vi "ProgressControl.vi"(0 "Elapsed time IN":dbl, 1 "SP IN":dbl, 2 "Array IN":dbl[](array[numeric]), 3 "Current SP IN":dbl, 4 "Stable":bool, 5 "Initial ramp IN":bool, 6 "SP reached IN":bool, 7 "Oven Watlows":refnum<visa-resource-name>="COM4", 8 "Progress":string, 9 "Sample":dbl) -> (12 "Array":dbl[](array[numeric]), 14 "Progress":string, 15 "Current SP":dbl, 16 "Stable":bool, 17 "Initial ramp":bool, 18 "SP reached":bool)   [LabVIEW 2009]
panel:
  # "INPUT"
  # "OUTPUT"
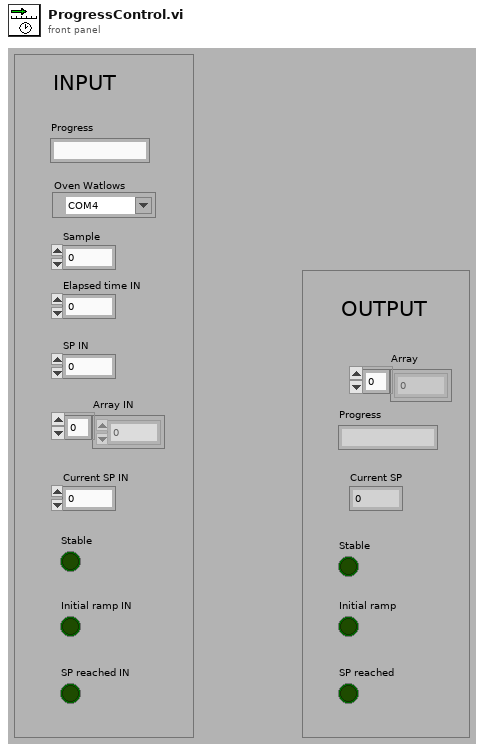
[diagram p1: front panel]
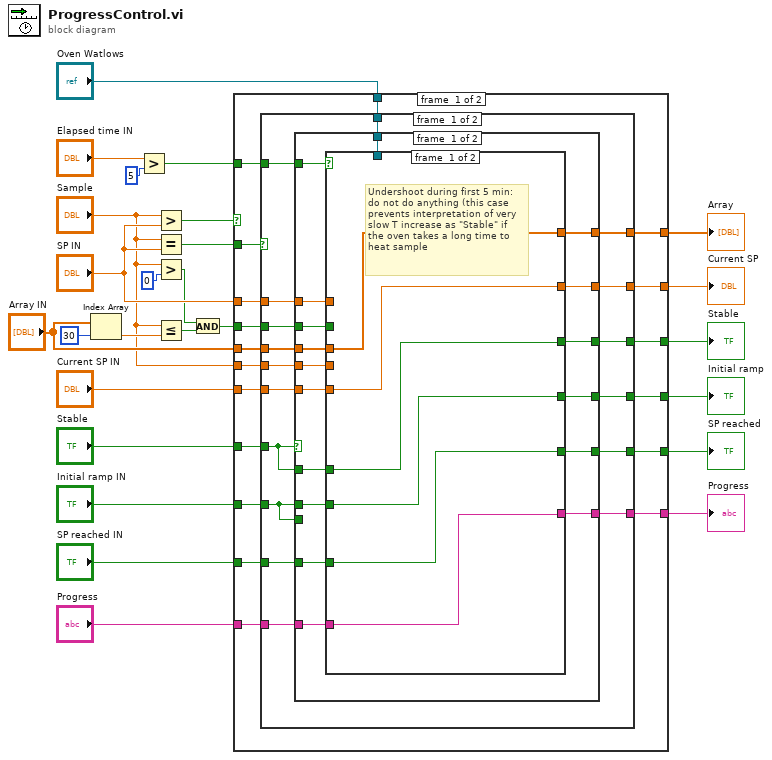
[diagram p0: block diagram]
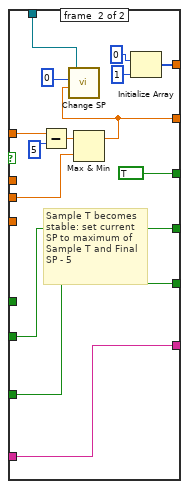
[diagram p3: hidden frame]
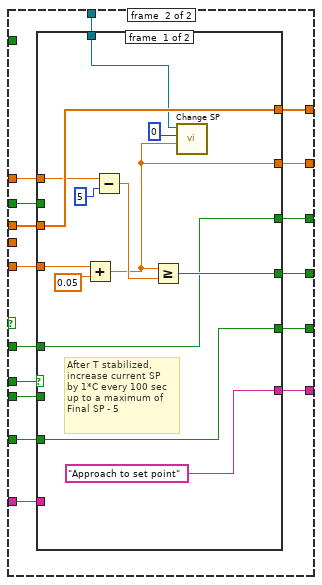
[diagram p4: hidden frame]
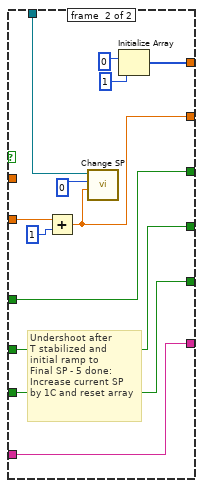
[diagram p6: hidden frame]
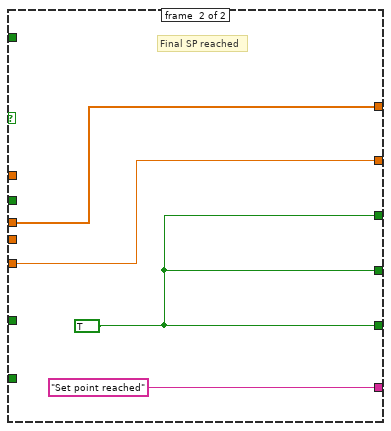
[diagram p7: hidden frame]
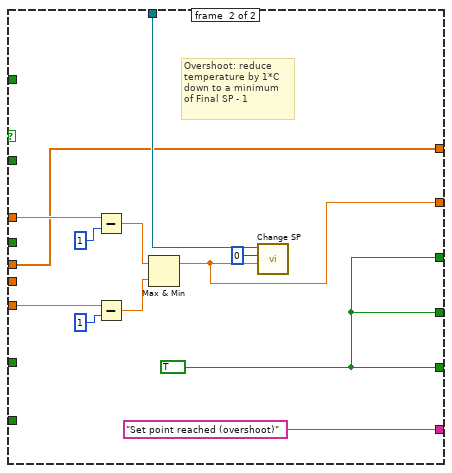
[diagram p8: hidden frame]
diagram:
  n1 = Index Array(array="Array IN", index=30) -> (element=w19:dbl)
  n2 = Greater?(x="Elapsed time IN", y=5) -> (0:w23:bool)
  n3 = Greater?(x="Sample", y="SP IN") -> (0:w6:bool)
  n4 = Equal?(x="Sample", y="SP IN") -> (x = y?=w7:bool)
  n5 = Greater?(x="Sample", y=0) -> (0:w1:bool)
  n6 = Less Or Equal?(x="Sample", y=w19) -> (x <= y?=w2:bool)
  n7 = And(x=w1, y=w2) -> (x .and. y?=w3:bool)
  n8 = case shown="False" w6 {
    tunnel: "SP reached IN" -> [w44 _]
    tunnel: w23 -> [w43 _]
    tunnel: w3 -> [w42 _]
    tunnel: "Oven Watlows" -> [w41 w188]
    tunnel: [w40 w187] -> w21
    tunnel: [w39 w186] -> w18
    tunnel: [w38 w197] -> w17
    tunnel: [w37 w197] -> w16
    tunnel: [w36 w197] -> w15
    tunnel: "Current SP IN" -> [w35 w194]
    tunnel: [w34 "Set point reached (overshoot)"] -> w13
    tunnel: "Stable" -> [w33 _]
    tunnel: "Initial ramp IN" -> [w32 _]
    tunnel: "Progress" -> [w31 _]
    tunnel: "Array IN" -> [w30 w186]
    tunnel: "Sample" -> [w29 _]
    tunnel: "SP IN" -> [w28 w191]
    tunnel: w7 -> [w27 _]
    frame #0 {
      n9 = case shown="False" w27 {
        tunnel: w44 -> [w61 _]
        tunnel: w43 -> [w60 _]
        tunnel: w42 -> [w59 _]
        tunnel: w41 -> [w58 _]
        tunnel: [w57 w183] -> w40
        tunnel: [w56 w184] -> w39
        tunnel: [w55 w182] -> w38
        tunnel: [w54 w182] -> w37
        tunnel: [w53 w182] -> w36
        tunnel: w35 -> [w52 w183]
        tunnel: [w51 "Set point reached"] -> w34
        tunnel: w33 -> [w50 _]
        tunnel: w32 -> [w49 _]
        tunnel: w31 -> [w48 _]
        tunnel: w30 -> [w47 w184]
        tunnel: w29 -> [w46 _]
        tunnel: w28 -> [w45 _]
        frame #0 {
          n10 = case shown="True" w50 {
            tunnel: w49 -> [w70 w136]
            tunnel: w61 -> [w68 w130]
            tunnel: w60 -> [w78 _]
            tunnel: w59 -> [w77 w125]
            tunnel: w46 -> [w76 _]
            tunnel: w58 -> [w75 w135]
            tunnel: [w74 w133] -> w57
            tunnel: [w73 w124] -> w56
            tunnel: [w72 w129] -> w55
            tunnel: [w71 w126] -> w54
            tunnel: [w69 w131] -> w53
            tunnel: w52 -> [w64 w134]
            tunnel: [w67 w132] -> w51
            tunnel: w50 -> [w63 w128]
            tunnel: w45 -> [w62 w127]
            tunnel: w49 -> [_ w123]
            tunnel: w48 -> [w66 w122]
            tunnel: w47 -> [w65 w121]
            frame #0 {
              n11 = case shown="True" w78 {
                tunnel: w77 -> [_ w100]
                tunnel: w76 -> [_ w98]
                tunnel: w75 -> [_ w92]
                tunnel: [w83 w90] -> w74
                tunnel: [w84 w91] -> w73
                tunnel: [w82 w89] -> w72
                tunnel: [w81 w88] -> w71
                tunnel: w70 -> [w81 w95]
                tunnel: [w80 w87] -> w69
                tunnel: w68 -> [w80 w94]
                tunnel: [w79 w86] -> w67
                tunnel: w66 -> [w79 w93]
                tunnel: w65 -> [w84 w99]
                tunnel: w64 -> [w83 w97]
                tunnel: w63 -> [w82 w96]
                tunnel: w62 -> [_ w85]
                frame #0 {
                  # "Undershoot during first 5 min:\ndo not do anything (this case\nprevents interpretation of very\nslow T increase as \"Stable\" if\nthe oven takes a long time to \nheat sample"
                }
                frame #1 {
                  n12 = case shown="True" w100 {
                    tunnel: w98 -> [_ w107]
                    tunnel: w92 -> [_ w119]
                    tunnel: [w105 w108] -> w90
                    tunnel: [w106 w116] -> w91
                    tunnel: [w104 TRUE] -> w89
                    tunnel: [w103 w114] -> w88
                    tunnel: w95 -> [w103 w114]
                    tunnel: [w102 w113] -> w87
                    tunnel: w94 -> [w102 w113]
                    tunnel: [w101 w112] -> w86
                    tunnel: w93 -> [w101 w112]
                    tunnel: w99 -> [w106 _]
                    tunnel: w97 -> [w105 _]
                    tunnel: w96 -> [w104 _]
                    tunnel: w85 -> [_ w110]
                    frame #0 {
                      # "Sample T not\nstable yet"
                    }
                    frame #1 {
                      # "Sample T becomes\nstable: set current\nSP to maximum of\nSample T and Final\nSP - 5"
                      n13 = Subtract(x=w110, y=5) -> (x-y=w109:dbl)
                      n14 = Max & Min(x=w109, y=w107) -> (max(x,y)=w108:dbl)  [unwired: 1 out]
                      n15 = call "Change SP.vi"("Set Point"=w108, "Adress"=0, "VISA resource name"=w119) -> ()  [unwired: 1 in, 1 out]
                      n16 = Initialize Array(0, 1) -> (w116:i32[])
                    }
                  }
                }
              }
            }
            frame #1 {
              n17 = case shown="True" w136 {
                tunnel: w135 -> [w142 w162]
                tunnel: w134 -> [w140 w161]
                tunnel: [w138 w160] -> w133
                tunnel: ["Approach to set point" w152] -> w132
                tunnel: [w148 w154] -> w131
                tunnel: w130 -> [w148 w153]
                tunnel: [w137 w158] -> w129
                tunnel: w128 -> [w137 w157]
                tunnel: w127 -> [w141 _]
                tunnel: [w139 w156] -> w126
                tunnel: w125 -> [_ w163]
                tunnel: [w147 w159] -> w124
                tunnel: w123 -> [_ w155]
                tunnel: w122 -> [_ w151]
                tunnel: w121 -> [w147 w150]
                frame #0 {
                  # "After T stabilized,\nincrease current SP\nby 1*C every 100 sec\nup to a maximum of \nFinal SP - 5"
                  n18 = Add(x=w140, y=0.05) -> (x+y=w138:dbl)
                  n19 = Subtract(x=w141, y=5) -> (x-y=w143:dbl)
                  n20 = Greater Or Equal?(x=w138, y=w143) -> (x >= y?=w139:bool)
                  n21 = call "Change SP.vi"("Set Point"=w138, "Adress"=0, "VISA resource name"=w142) -> ()  [unwired: 1 in, 1 out]
                }
                frame #1 {
                  n22 = case shown="False" w163 {
                    tunnel: w162 -> [_ w172]
                    tunnel: w161 -> [w168 w171]
                    tunnel: [w168 w170] -> w160
                    tunnel: [w169 w173] -> w159
                    tunnel: [w167 w178] -> w158
                    tunnel: w157 -> [w167 w178]
                    tunnel: [w166 w179] -> w156
                    tunnel: w155 -> [w166 w179]
                    tunnel: [w165 w180] -> w154
                    tunnel: w153 -> [w165 w180]
                    tunnel: [w164 w181] -> w152
                    tunnel: w151 -> [w164 w181]
                    tunnel: w150 -> [w169 _]
                    frame #0 {
                      # "Default case:\noccurs when\nWatlow read\nerror (Sample\nT = 0), and \nwhen T has\nnot stabilized\nafter change"
                    }
                    frame #1 {
                      # "Undershoot after\nT stabilized and\ninitial ramp to \nFinal SP - 5 done:\nIncrease current SP\nby 1C and reset array"
                      n23 = Add(x=w171, y=1) -> (x+y=w170:dbl)
                      n24 = call "Change SP.vi"("Set Point"=w170, "Adress"=0, "VISA resource name"=w172) -> ()  [unwired: 1 in, 1 out]
                      n25 = Initialize Array(0, 1) -> (w173:i32[])
                    }
                  }
                }
              }
            }
          }
        }
        frame #1 {
          w182 = TRUE
          # "Final SP reached"
        }
      }
    }
    frame #1 {
      w197 = TRUE
      # "Overshoot: reduce\ntemperature by 1*C\ndown to a minimum\nof Final SP - 1"
      n26 = Subtract(x=w191, y=1) -> (x-y=w190:dbl)
      n27 = Subtract(x=w194, y=1) -> (x-y=w193:dbl)
      n28 = Max & Min(x=w190, y=w193) -> (max(x,y)=w187:dbl)  [unwired: 1 out]
      n29 = call "Change SP.vi"("Set Point"=w187, "Adress"=0, "VISA resource name"=w188) -> ()  [unwired: 1 in, 1 out]
    }
  }
  "Stable" <- w17
  "Initial ramp" <- w16
  "SP reached" <- w15
  "Current SP" <- w21
  "Progress" <- w13
  "Array" <- w18
